vi "ResetStat.vi"   [LabVIEW 2017]
uses:
  Global_SNK3_HF.vi
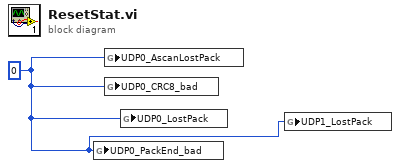
[diagram p0: block diagram]
diagram:
  w1 = u32 0 ("UDP0_AscanLostPack")
  n1 = global write "Global_SNK3_HF.vi" "UDP0_PackEnd_bad"(w1) -> ()
  n2 = global write "Global_SNK3_HF.vi" "UDP0_AscanLostPack"(w1) -> ()
  n3 = global write "Global_SNK3_HF.vi" "UDP0_CRC8_bad"(w1) -> ()
  n4 = global write "Global_SNK3_HF.vi" "UDP0_LostPack"(w1) -> ()
  n5 = global write "Global_SNK3_HF.vi" "UDP1_LostPack"(w1) -> ()
